vi "manual_ws_conn.vi"() -> ()   [LabVIEW 2013]
uses:
  <vilib>/Intelligent Energy/WebSockets API/WebSockets/WebSockets.lvlib
panel:
  out "Data":string
  in  "stop":bool
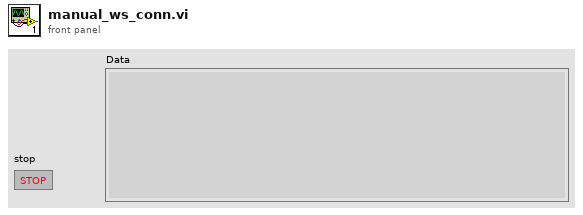
[diagram p1: front panel]
types:
  T1 = enum16{"Standard", "Buffered", "CRLF", "Immediate"}
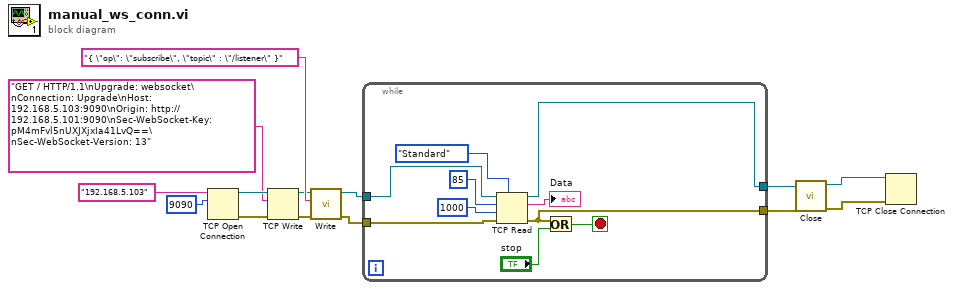
[diagram p0: block diagram]
diagram:
  n1 = TCP Open Connection(address="192.168.5.103", remote port or service name=u16 9090) -> (connection ID=w12:refnum<k5>, error out=w10:errorcluster)  [unwired: 3 in]
  n2 = TCP Write(connection ID=w12, data in="GET / HTTP/1.1\nUpgrade: websocket\nConnection: Upgrade\nHost: 192.168.5.103:9090\nOrigin: http://192.168.5.101:9090\nSec-WebSocket-Key: pM4mFvl5nUXJXjxIa41LvQ==\nSec-WebSocket-Version: 13", error in (no error)=w10) -> (connection ID out=w6:refnum<k5>, error out=w5:errorcluster)  [unwired: 1 in, 1 out]
  n3 = call <vilib>:"Write.vi"("error in (no error)"=w5, "Data"="{ \"op\": \"subscribe\", \"topic\" : \"/listener\" }", "WebSocket Connection in"=w6) -> ("error out"=w1:errorcluster, "WebSocket Connection out"=w2:refnum<k5>)  [unwired: 7 in]
  n4 = while {
    tunnel: [w21] -> w4
    tunnel: [w20] -> w3
    tunnel: w2 -> [w22]
    tunnel: w1 -> [w15]
    stop <- w24 stop-if-true
    n5 = TCP Read(connection ID=w22, bytes to read=85, error in (no error)=w15, 7:T1."Standard" ("mode (standard)"), 9:1000 ("timeout ms (25000)")) -> (connection ID out=w21:refnum<k5>, data out=→"Data":string, error out=w20:errorcluster)
    n6 = Or(x=w20, y="stop") -> (x .or. y?=w24:bool)
  }
  n7 = call <vilib>:"Close.vi"("error in (no error)"=w3, "WebSocket Connection in"=w4) -> ("error out"=w7:errorcluster, "WebSocket Connection in"=w8:refnum<k5>)  [unwired: 8 in]
  n8 = TCP Close Connection(connection ID=w8, error in (no error)=w7) -> ()  [unwired: 1 in, 2 out]
